vi "To String.vi"(8 "error in (no error)":errorcluster, 11 "Types in":refnum<class "Abs_String.lvclass">) -> (0 "error out":errorcluster, 2 "String":string, 3 "Types out":refnum<class "Abs_String.lvclass">)   [LabVIEW 2021, in "Abs_String.lvclass"]
uses:
  Abs_String.lvclass
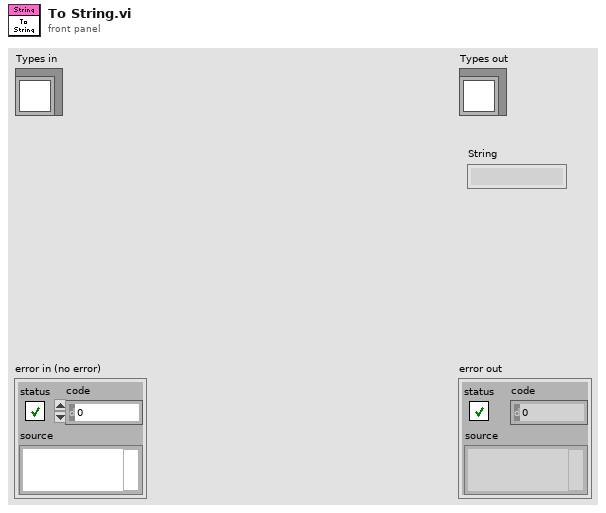
[diagram p1: front panel]
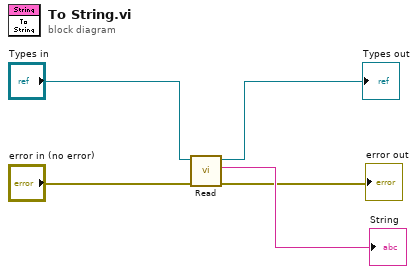
[diagram p0: block diagram]
diagram:
  n1 = call-dynamic "Read.vi"("error in (no error)"="error in (no error)", "Abs_String in"="Types in") -> ("error out"=→"error out":errorcluster, "String"=→"String":string, "Abs_String out"=→"Types out":refnum<class "Abs_String.lvclass">)  [unwired: 7 in]
